vi "Config Dev Rolloff.vi"(8 "error in":errorcluster, 10 "Rolloff Point (3000 Hz)":dbl=3000.0 min=0.0003 max=4200.0, 11 "VISA resource name":refnum<visa-resource-name>) -> (0 "error out":errorcluster, 3 "VISA resource name out":refnum<visa-resource-name>)   [LabVIEW 2017, in "Andeen-Hagerling 2700.lvlib"]
doc: "This VI sets the 3 db down point of the analog output frequency roll off limit.\n\nEven though the highest permissible value for DRolloff is 4200 Hz, the highest achievable 3 db frequency\nDRolloffMax is given by the following expression: DRolloffMax = 0.3 * Minimum( Freq, 28 kHz - Freq )\nwhere Freq is the bridge frequency in Hz."
uses:
  Andeen-Hagerling 2700.lvlib
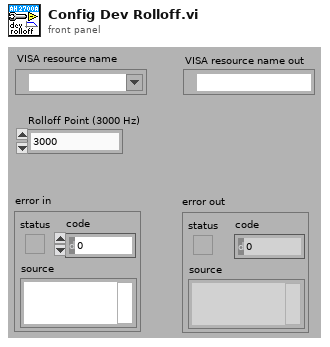
[diagram p1: front panel]
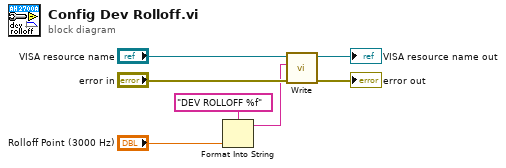
[diagram p0: block diagram]
diagram:
  n1 = Format Into String(format string="DEV ROLLOFF %f", "Rolloff Point (3000 Hz)") -> (resulting string=w2:string)  [unwired: 2 in, 1 out]
  n2 = call "Write.vi"("error in"="error in", "command"=w2, "VISA resource name"="VISA resource name") -> ("error out"=→"error out":errorcluster, "VISA resource name out"=→"VISA resource name out":refnum<visa-resource-name>)  [unwired: 7 in]
